vi "Write Active Frame.vi"(5 "Active Frame":i16, 9 "DiagramDisable in":refnum<class "DiagramDisable.lvclass">) -> (3 "DiagramDisable out":refnum<class "DiagramDisable.lvclass">)   [LabVIEW 2014, in "Raspberry Pi Compatible Compiler for LabVIEW.lvlib" / "DiagramDisable.lvclass"]
uses:
  DiagramDisable.lvclass
  DiagramDisable.lvclass/DiagramDisable.ctl
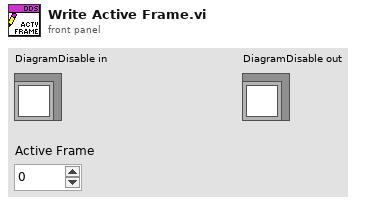
[diagram p1: front panel]
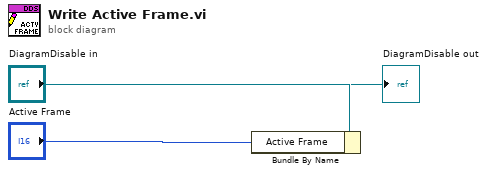
[diagram p0: block diagram]
diagram:
  n1 = Bundle By Name(cluster="DiagramDisable in", "Active Frame"="Active Frame") -> (→"DiagramDisable out":refnum<class "DiagramDisable.lvclass">)
